vi "Dashboard Main.vi"() -> ()   [LabVIEW 2016]
uses:
  <vilib>/Rock Robotics/WPI/Camera/WPI_CameraExposure Values.ctl
  <vilib>/Rock Robotics/WPI/Camera/WPI_CameraWhite Balance Values.ctl
  <vilib>/Utility/miscctls.llb/LVRowAndColumnTypeDef.ctl
  <vilib>/event_ctls.llb/eventvkey.ctl
  <vilib>/Rock Robotics/Network Tables/NT Read Numeric Array.vi
  <vilib>/Rock Robotics/WPI/Dashboard/WPI_DashboardLogging Global.vi
  <vilib>/vision/NI_Vision_Development_Module.lvlib
panel:
  in  "Camera Settings 2":T3={"Exposure"=enum."Custom", "Exposure (%)"=0.0, "Brightness"=0, "White Balance"=enum."Custom", "Color Temp (K)"=0.0}
  out "Particle Reports (Pixels)":T4(array[cluster]) {"Orientation" format="%.2f"; "Dimensions"."Height" format="%.2f"; "Dimensions"."Width" format="%.2f"; "Center of Mass"."Y" format="%.2f"; "Center of Mass"."X" format="%.2f"; "Bounding Rect"."Bottom" format="%.2f"; "Bounding Rect"."Right" format="%.2f"; "Bounding Rect"."Top" format="%.2f"; "Bounding Rect"."Left" format="%.2f"; "Number of Holes" format="%.2f"; "Area" format="%.2f"}
  out "Detected and good":bool
  in  "Camera Settings Right":T5={"Frame Rate"=30, "Compression"=30, "Size"=1, "DB Camera Config"=FALSE} {"Frame Rate" scale=1.0..30.0; "Compression" scale=100.0..-1.0; "Size" items=["640x480", "320x240", "160x120"]}
  in  "Camera Name Right":string(combo)="No Camera Selection"
  out "Camera Info":cluster{"Mbps LED":bool, "Mbps":dbl, "fps":dbl} {"fps" format="%#.1g"; "Mbps" format="%#.1g"}
  in  "Camera Settings":T5={"Frame Rate"=30, "Compression"=30, "Size"=1, "DB Camera Config"=FALSE} {"Frame Rate" scale=1.0..30.0; "Compression" scale=100.0..-1.0; "Size" items=["640x480", "320x240", "160x120"]}
  in  "TCP":refnum<k5>
  in  "Rec Mode":enum32{"Stop", "Record", "Playback"}(radio)
  out "Robot IP":string
  out "Image Message":string="Timeout in Camera Communications"
  in  "Dashboard Tab":T6(tab)
  in  "Select Auto":string(combo)="Select Autonomous ..."
  out "NT Connection":bool
  out "MotorChart R":cluster{"Numeric":dbl, "Numeric":dbl}(graph)
  out "MotorChart L":cluster{"Numeric":dbl, "Numeric":dbl}(graph)
  out "MotorSliders R":cluster{"MotorSlide1":dbl, "MotorSlide2":dbl} {"MotorSlide2" scale=-1.0..1.0 scale format="%#_2e"; "MotorSlide1" scale=-1.0..1.0 scale format="%#_2e"}
  out "MotorSliders L":cluster{"MotorSlide1":dbl, "MotorSlide2":dbl} {"MotorSlide2" scale=-1.0..1.0 scale format="%#_2e"; "MotorSlide1" scale=-1.0..1.0 scale format="%#_2e"}
  out "Gyro":dbl(knob) scale=0.0..360.0
  out "JS1 Z":dbl(slide) scale=-1.0..1.0 scale format="%#_2e"
  out "JS1 Graph":cluster{"X":dbl, "Y":dbl}[](graph)
  out "JS1 Buttons":T7
  out "JS2 Z":dbl(slide) scale=-1.0..1.0 scale format="%#_2e"
  out "JS2 Graph":cluster{"X":dbl, "Y":dbl}[](graph)
  out "JS2 Buttons":T7
  out "Mode":T8(ring)=enum."Auto Disabled"
  in  "Observer Gain":dbl=0.5
  out "Detected":bool
  out "Camera Image Right":T9(plugin-control)
  in  "DB/String 9":string
  in  "DB/String 8":string
  in  "DB/String 7":string
  in  "DB/String 6":string
  in  "DB/String 5":string
  in  "DB/String 4":string
  in  "DB/String 3":string
  in  "DB/String 2":string
  in  "DB/String 1":string
  in  "DB/String 0":string
  in  "DB/Slider 0":dbl(slide) scale=0.0..5.0
  in  "DB/Slider 1":dbl(slide) scale=0.0..5.0
  in  "DB/Slider 2":dbl(slide) scale=0.0..5.0
  in  "DB/Slider 3":dbl(slide) scale=0.0..5.0
  out "DB/LED 3":bool
  out "DB/LED 2":bool
  out "DB/LED 1":bool
  out "DB/LED 0":bool
  in  "DB/Button 3":bool
  in  "DB/Button 2":bool
  in  "DB/Button 1":bool
  in  "DB/Button 0":bool caption="New Name"
  in  "Test Slider":dbl(slide) scale=0.0..100.0 scale format="%#_3g"
  in  "On/Off":bool caption="Solenoid"
  in  "Test Name":u16(ring) items=["Select the test to run..."]
  in  "Test Tree":string(tree)
  in  "Motor":cluster{"Value":dbl, "Enable":bool} {"Value" scale=-1.0..1.0 scale format="%#_3g"}
  out "Progress":T10 {"Test Progress" scale=0.0..100.0}
  in  "Rev/Fwd":cluster{"Forward":bool, "Reverse":bool}
  in  "Test Ring":u16(ring) items=["Monochrome", "Color"]
  out "Cmd Status":string
  in  "Execute Command":bool
  in  "Command Params":string[][](table)
  in  "Command Selection":i32(listbox)
  in  "CheckList":i32(listbox)
  out "Tree":string(tree)
  out "Camera Image":T9(plugin-control)
  out "Background":bool
  in  "Camera Name":string(combo)="Camera"
  # "HW"
  # "HW"
  # "Joysticks"
  # "Drive Motors"
  # "Front"
  # "Right"
  # "Left"
  # "Back"
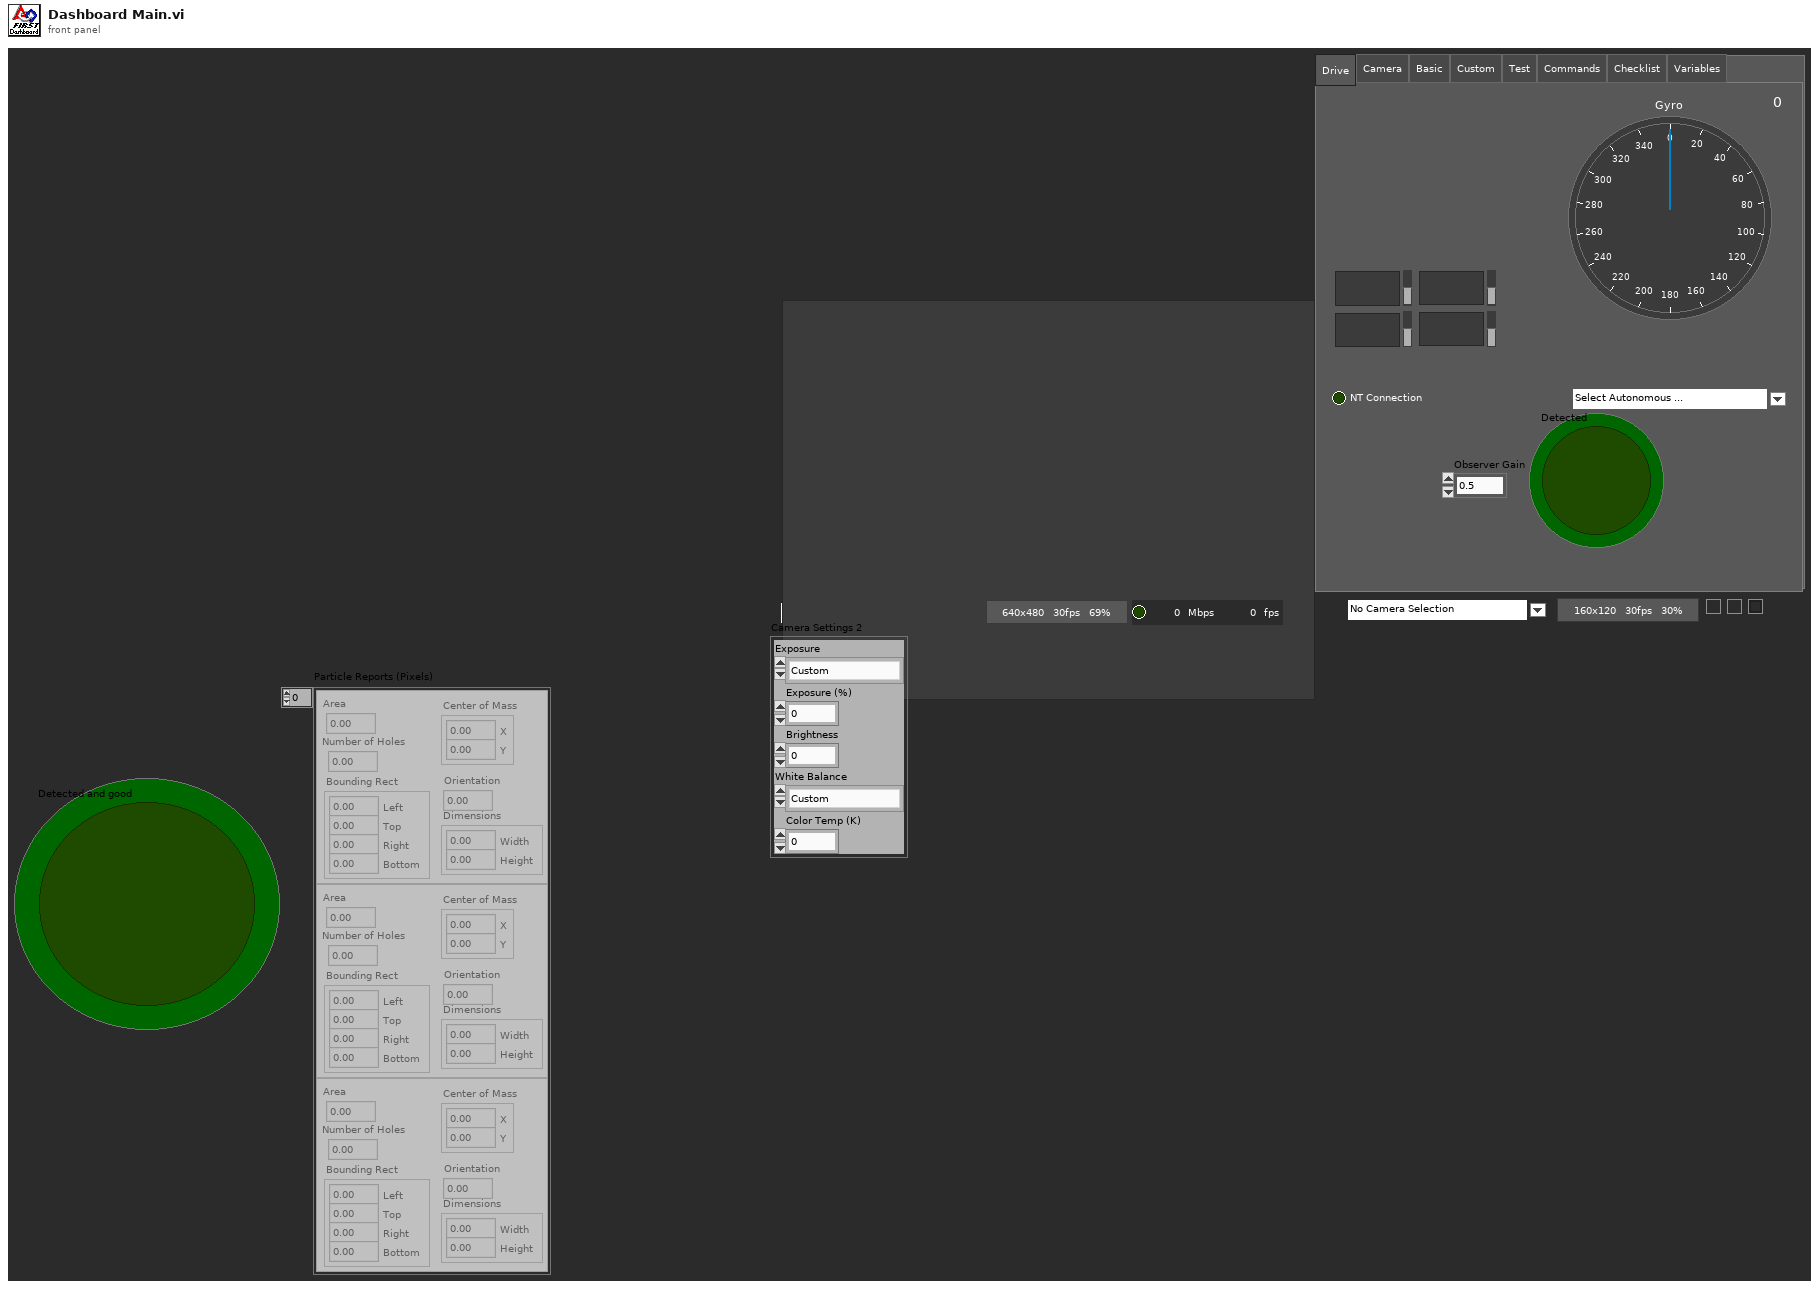
[diagram p1: front panel]
types:
  T1 = typedef "WPI_CameraExposure Values.ctl" = enum16{"Auto", "Flicker-free 50 Hz", "Flicker-free 60 Hz", "Hold current", "Custom"}
  T2 = typedef "WPI_CameraWhite Balance Values.ctl" = enum16{"Auto", "Fixed indoor", "Fixed outdoor 1", "Fixed outdoor 2", "Fixed fluorescent 1", "Fixed fluorescent 2", "Hold current", "Custom"}
  T3 = cluster{"Exposure":T1, "Exposure (%)":dbl, "Brightness":i32, "White Balance":T2, "Color Temp (K)":dbl}
  T4 = cluster{"Area":dbl, "Number of Holes":dbl, "Bounding Rect":cluster{"Left":dbl, "Top":dbl, "Right":dbl, "Bottom":dbl}, "Center of Mass":cluster{"X":dbl, "Y":dbl}, "Orientation":dbl, "Dimensions":cluster{"Width":dbl, "Height":dbl}}[]
  T5 = cluster{"Frame Rate":i32, "Compression":i32, "Size":u16, "DB Camera Config":bool}
  T6 = enum32{"Drive", "Camera", "Basic", "Custom", "Test", "Commands", "Checklist", "Variables"}
  T7 = cluster{bool, bool, bool, bool, bool, bool, bool, bool, bool, bool, bool, bool}
  T8 = enum8{"Tele-Op Disabled", "Tele-Op Enabled", "Auto Disabled", "Auto Enabled", "Test Disabled", "Test Enabled", "Disconnected", "No Code", "E-Stop"}
  T9 = typedef "IMAQ Image.ctl" = refnum<image>
  T10 = cluster{"Test Progress":u8, "Test Progress Text":string}
  T11 = typedef "Image Type" = u32
  T12 = cluster{"IDs":cluster{"RPC field ID":u16, "Unique ID":u16}, "String":string}
  T13 = enum32{"Drive", "Basic", "Custom", "Test", "Checklist", "Variables"}
  T14 = cluster{"Camera Image":refnum<vi>, "Dashboard Tab":refnum<vi>, "Background":refnum<vi>, "Rec Mode":refnum<vi>, "Test Slider":refnum<vi>, "On/Off ":refnum<vi>, "Test Ring":refnum<vi>, "Rev/Fwd":refnum<vi>, "Test Name":refnum<vi>, "Motor":refnum<vi>, "Progress":refnum<vi>, "CheckList":refnum<vi>, "Tree":refnum<vi>, "Test Tree":refnum<vi>, "Command Params":refnum<vi>, "Command Selection":refnum<vi>, "Execute Command":refnum<vi>, "Cmd Status":refnum<vi>, "Camera Settings":refnum<vi>, "Camera Name":refnum<vi>, "Camera Info":refnum<vi>, "Camera Settings Right":refnum<vi>, "Camera Name Right":refnum<vi>, "Camera Image Right":refnum<vi>}
  T15 = cluster{"Error Strings":string, "Disable Counts":cluster{u16, u16}, "Rail Faults":cluster{u16, u16, u16}, "Robot IP":string, "DB Mode":u8, "Event Info":cluster{"Name":string, "Type":u8, "Number":u16, "Replay":u8}}
  T16 = cluster{"Storage":cluster{"Disk Free":u64, "RAM Block":u32, "RAM free":u32}, "CPU Utilization":cluster{"CPU % ISR":sgl, "CPU % Time Crit":sgl, "CPU % Timed Str":sgl, "CPU % High":sgl, "CPU % Above":sgl, "CPU % Normal":sgl, "CPU % Low":sgl}, "CAN":cluster{"% Bus Utilization":sgl, "Bus Off Cnt":u32, "TX_FIFO Full Cnt":u32, "Receive Error Cnt":u8, "Transmit Error Cnt":u8}, "HID":cluster{"HID Outputs":u32, "Rumble Low":u16, "Rumble High":u16}[]}
  T17 = cluster{"Status bits":cluster{"Test Mode":bool, "Autonomous":bool, "Enabled":bool, "Code Start":bool, "Brownout":bool, "Reserved 2":bool, "Reserved 3":bool, "E-Stop":bool}, "Code Trace":cluster{"Disabled":bool, "TeleOp":bool, "Auto":bool, "Test":bool}, "Controller Type":enum16{"unknown", "cRIO", "roboRio"}, "Code?":enum16{"unknown", "noCode", "code"}, "Battery V":dbl}
  T18 = cluster{"Control Bits":cluster{"TestMode":bool, "Autonomous":bool, "Enabled":bool, "FMS Present":bool, bool, bool, bool, "E-Stop":bool}, "Team Station ":u8, "Countdown":sgl, "Joystick Values":cluster{"Axes":dbl[], "Buttons":bool[], "POVs":i16[]}[]}
  T19 = cluster{"Axes":dbl[], "Buttons":bool[], "POVs":i16[]}[]
  T20 = cluster{"Axes":dbl[], "Buttons":bool[], "POVs":i16[]}
  T21 = cluster{"Buttons[0]":bool, "Buttons[1]":bool, "Buttons[2]":bool, "Buttons[3]":bool, "Buttons[4]":bool, "Buttons[5]":bool, "Buttons[6]":bool, "Buttons[7]":bool, "Buttons[8]":bool, "Buttons[9]":bool, "Buttons[10]":bool, "Buttons[11]":bool}
  T22 = cluster{"Operation":enum16{"Update", "Clear"}, "Color Box":u32}[]
  T23 = typedef "eventvkey.ctl" = enum16{"ASCII", "Enter", "Return", "Shift", "Ctrl", "Alt", "Cmd", "Opt", "Caps", "NumLock", "Clear", "Break", "Up", "Down", "Left", "Right", "Insert", "Delete", "Home", "End", "PageUp", "PageDown", "Escape", "Help", "Pause", "ScrollLock", "F1", "F2", "F3", "F4", "F5", "F6", "F7", "F8", "F9", "F10", "F11", "F12", "F13", "F14", "F15", "F16", "F17", "F18", "F19", "F20", "F21", "F22", "F23", "F24", "Play", "VolumeUp", "VolumeDown", "Mute", "Two Byte Char"}
  T24 = cluster{"Image Size":bool, "Image Type":bool, "Pixel Value":bool, "ROI Information":bool, "Zoom Factor":bool}
  T25 = cluster{"Operation":enum16{"Update", "Clear"}, "Color Box":u32}
  T26 = typedef "LVRowAndColumnTypeDef.ctl" = cluster{"Row":i32, "Column":i32}
  T27 = cluster{"Shift":bool, "Ctrl":bool, "Alt":bool, "Cmd":bool, "Opt":bool}
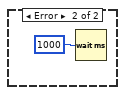
[diagram p3: hidden frame]
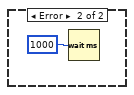
[diagram p4: hidden frame]
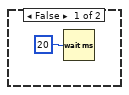
[diagram p5: hidden frame]
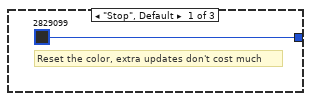
[diagram p6: hidden frame]
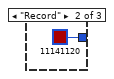
[diagram p7: hidden frame]
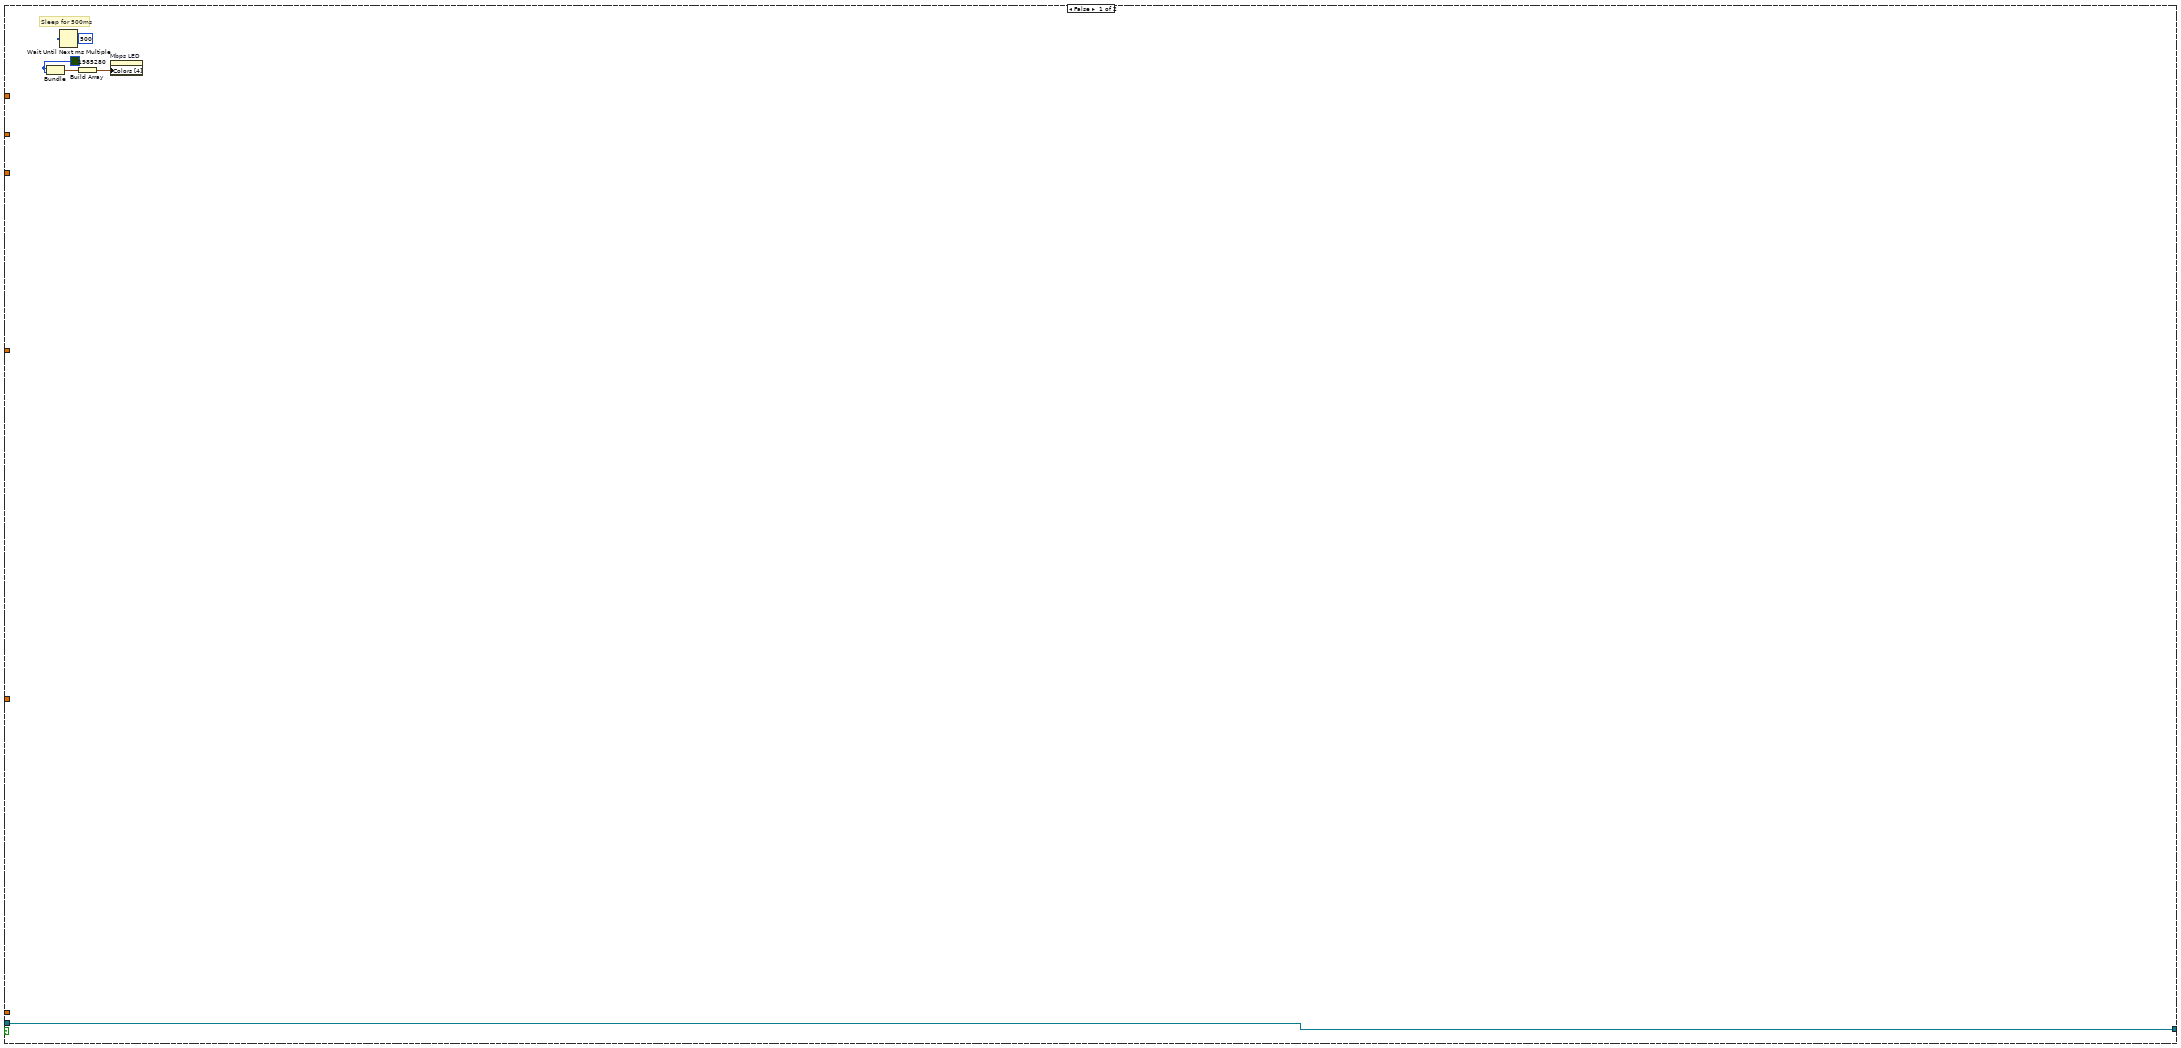
[diagram p9: hidden frame]
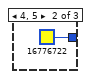
[diagram p11: hidden frame]
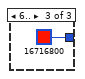
[diagram p12: hidden frame]
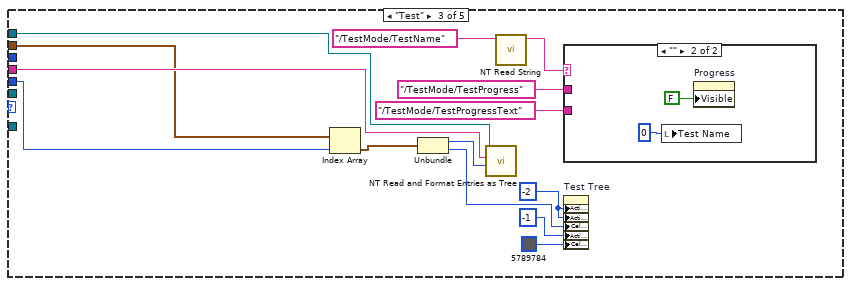
[diagram p14: hidden frame]
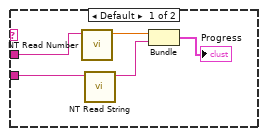
[diagram p15: hidden frame]
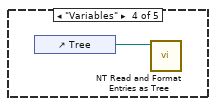
[diagram p16: hidden frame]
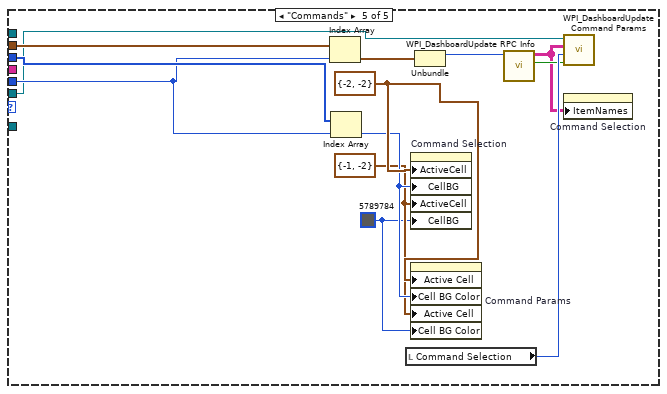
[diagram p17: hidden frame]
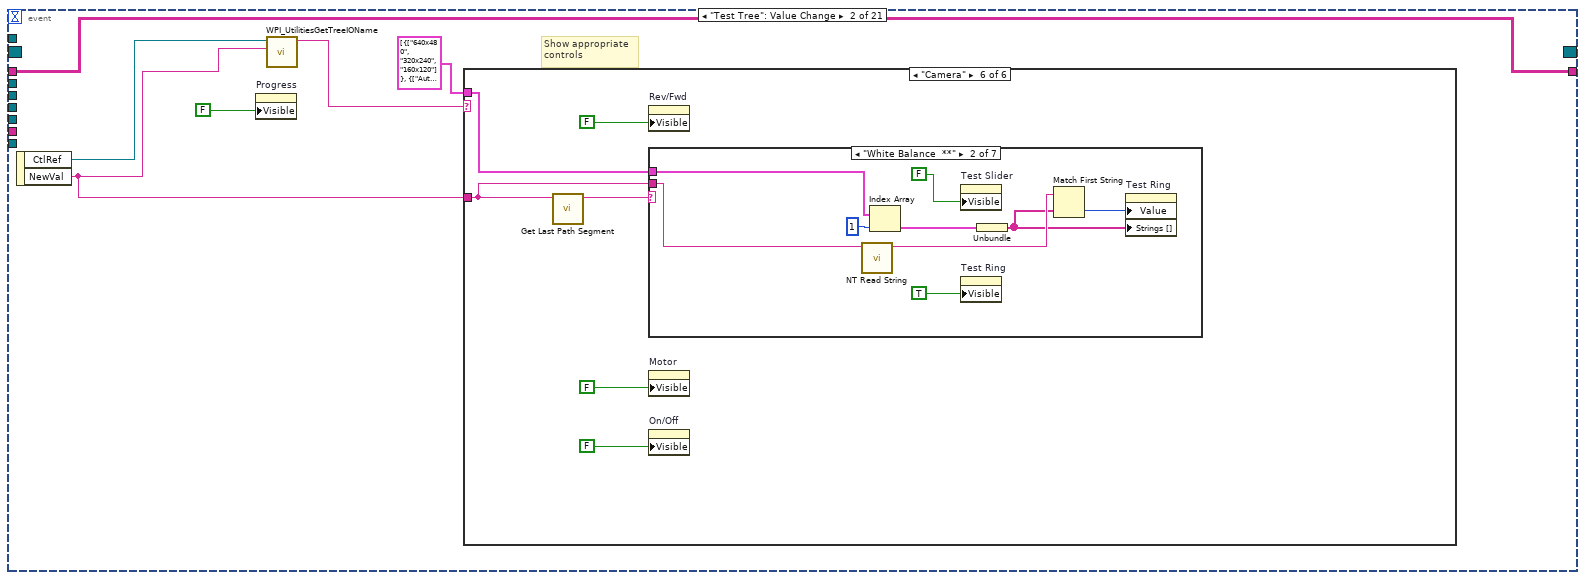
[diagram p18: hidden frame]
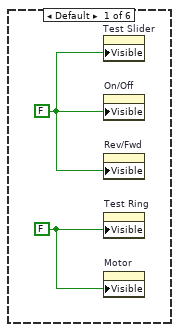
[diagram p19: hidden frame]
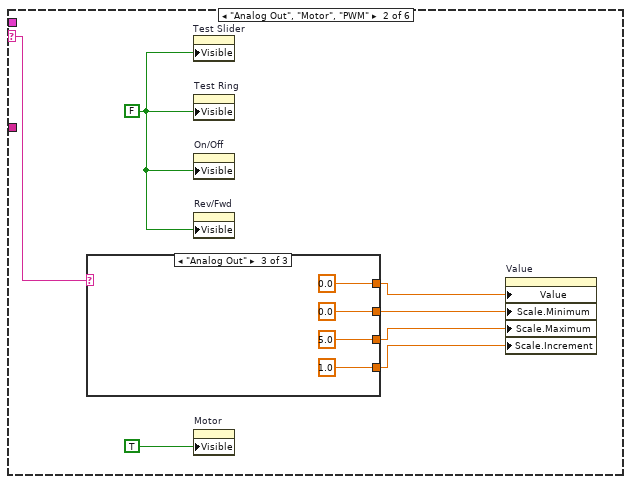
[diagram p20: hidden frame]
diagram:
  w10 = T11 4 items=["Grayscale (U8)", "Grayscale (I16)", "Grayscale (SGL)", "Complex (CSG)", "RGB (U32)", "HSL (U32)", "RGB (U64)"] ("Image Type")
  w26 = T12 {"IDs"={"RPC field ID"=0, "Unique ID"=0}, "String"=""}  # RPC Response
  w51 = 491  # min tab size
  w50 = 1.333  # min tab size
  w58 = enum32{"Stop", "Record", "Playback"}."Stop" ("Rec Mode")
  w33 = FALSE ("Visible")
  (unwired) "This VI has seven parallel loops for different tasks and a bit of initialization code that runs just once.\n\nTypical dashboard extensions only need to edit the panel. Adding new indicators or controls simply involves placing them on the panel in the Operations tab and naming them the same as the SmartDashboard variable on the robot\n\nIf the display needs to process the data before display, loop one is an example of doing that for the joysticks and motors.\n\nIf you want customize the video display or perform processing on it, loop two is where that takes place.\n\nOther loops should not need to be modified. They are pretty standard, and document the task they perform."  # Documentation
  w75 = T11 4 items=["Grayscale (U8)", "Grayscale (I16)", "Grayscale (SGL)", "Complex (CSG)", "RGB (U32)", "HSL (U32)", "RGB (U64)"] ("Image Type")
  # "Loop 2.5 Receive additional camera images from robot and display"
  # "Command Param Info"
  # "Started one, Unique ID holds\nresponse"
  # "Loop 7. Wait for DS connections"
  # "Basic debug and auto controls: Their data names are fixed, but\nthe displayed name, called a caption, can be changed directly or in\nrobot code such as shown in Begin."
  # "Controls for Test Mode, Camera Settings, etc."
  # "Additional UI Initialization"
  # "Loop 6. Animation for background of window during playback and record"
  # "Fires each time robot IP\nchanges, simulator does this"
  # "Fires each time window\ndocking changes."
  # "Collects all controls and indicators\nin the Basic and Custom tab.\nIf you need to bind additional controls,\nadd their references. You can extend the\nenum constant or use an integer."
  # "The remaining code below this line typically doesn't need to be modified."
  # "Loop 4. Process UI events related to test mode, checklist, and camera settings"
  # "Terminals of controls and indicators that are bound to the smart dashboard by name.\nYou can place the terminals anywhere you like and even read data from them.\nYou bind controls by adding the control reference to the array on the left. The subVI will\ndo this for the contents of a tab, and you can do it for individual items too, as shown with\nthe LED. To create get the reference, right-click and Create>>Reference."
  # "Loop 3. Wait until the robot response provides\n the Robot IP address.\nOnce known, bind controls and\nvariables with the same names."
  # "Loop 5. Adjusts placement onscreen, hides the titlebar, etc."
  # "Loop 1. Receive various data streams from Driver Station, update joystick, motors, and more complex displays that don't easily bind to variables."
  # "Loop 2. Receive camera images from robot, update Mbps, fps, and do any processing or display"
  n1 = control-ref of="Camera Settings"() -> (w19:refnum<vi>)
  n2 = control-ref of="Camera Name Right"() -> (w6:refnum<vi>)
  n3 = property class="VI"() -> ("Panel"=w65:refnum<vi>)  [unwired: 2 in, 2 out]
  n4 = control-ref of="Camera Name"() -> (w18:refnum<vi>)
  n5 = local write "Command Selection"(u16 0 ("milliseconds to wait")) -> ()
  n6 = property on="On/Off" class="Bool (strict)"("Visible"=w33) -> ()  [unwired: 2 in, 2 out]
  n7 = property on="Rev/Fwd" class="Clust (strict)"("Visible"=w33) -> ()  [unwired: 2 in, 2 out]
  n8 = property on="Motor" class="Clust (strict)"("Visible"=w33) -> ()  [unwired: 2 in, 2 out]
  n9 = property on="Progress" class="Clust (strict)"("Visible"=w33) -> ()  [unwired: 2 in, 2 out]
  n10 = property on="Test Ring" class="Ring (strict)"("Visible"=w33) -> ()  [unwired: 2 in, 2 out]
  n11 = while {
    tunnel: u16 1741 ("timeout ms (25000)") -> [w77]
    stop <- FALSE stop-if-true
    n12 = TCP Create Listener(10:w77) -> (0:w76:errorcluster, 3:w78:refnum<k5>)  [unwired: 4 in, 1 out]
    n13 = case shown="No Error" w76 {
      selector: w76 -> [w80 _]
      tunnel: w78 -> [w81 _]
      frame No Error {
        n14 = while {
          tunnel: w81 -> [w84]
          tunnel: w80 -> [w83]
          stop <- FALSE stop-if-true
          n15 = TCP Wait On Listener(8:w83, 11:w84) -> (0:w85:errorcluster, 4:w86:refnum<k5>)  [unwired: 2 in, 3 out]
          n16 = case shown="No Error" w85 {
            frame No Error {
            }
            frame Error {
              n17 = Wait (ms)(milliseconds to wait=u32 1000) -> ()  [unwired: 1 out]
            }
          }
          n18 = local write "TCP"(w86) -> ()
        }
      }
      frame Error {
        n19 = Wait (ms)(milliseconds to wait=u32 1000) -> ()  [unwired: 1 out]
      }
    }
  }
  n20 = local write "Rec Mode"(w58) -> ()
  n21 = global write "WPI_DashboardLogging Global.vi" "Recording"(w58) -> ()
  n22 = property class="Pnl"(reference=w65) -> ("Panes[]"=w66:refnum<vi>[])  [unwired: 1 in, 2 out]
  n23 = local write "Command Params"(string[][] [] ("Command Params")) -> ()
  n24 = local write "Dashboard Tab"(T6."Drive" ("Dashboard Tab")) -> ()
  n25 = call "Handle Camera Configuration.vi"("CameraNameRef"=w18, "Camera File Name"="Left", "ClusterRef"=w19) -> ()  [unwired: 9 in]
  n26 = call "IMAQ Create"("Image Name"="Dashboard Image", "Image Type"=w75) -> ("New Image"=w73:T9, "error out"=w72:errorcluster)  [unwired: 2 in, 1 out]
  n27 = Index Array(array=w66) -> (element=w64:refnum<vi>)  [unwired: 1 in]
  n28 = call "IMAQ Create"("Image Name"="Dashboard ImageRight", "Image Type"=w10) -> ("New Image"=w9:T9, "error out"=w8:errorcluster)  [unwired: 2 in, 1 out]
  n29 = while {
    tunnel: w73 -> [w95]
    tunnel: w72 -> [_]
    tunnel: [w96] -> _
    i -> [w96]
    stop <- FALSE stop-if-true
    n30 = flat-sequence {
      tunnel: w95 -> [w104]
      tunnel: [w104] -> w94
      tunnel: [w102] -> w93
      tunnel: [w98] -> w92
      tunnel: [w99] -> w91
      tunnel: [w99] -> w90
      tunnel: [w98] -> w89
      tunnel: w94 -> [w120]
      tunnel: w93 -> [w111]
      tunnel: w92 -> [w110]
      tunnel: w91 -> [w109]
      tunnel: w90 -> [w108]
      tunnel: w89 -> [w107]
      frame #0 {
        n31 = call-poly <vilib>:"NT Read Value.vi"("Name"="Y Latency") -> ("Numeric"=w99:dbl)  [unwired: 9 in, 1 out]
        n32 = call-poly <vilib>:"NT Read Value.vi"("Name"="X Latency") -> ("Numeric"=w98:dbl)  [unwired: 9 in, 1 out]
        n33 = call-poly <vilib>:"NT Read Value.vi"("Name"="Navx Yaw Latency") -> ("Numeric"=w102:dbl)  [unwired: 9 in, 1 out]
      }
      frame #1 {
        # "Optionally read the DB image,\nlog, or retrieve images from a\nlogged match"
        n34 = local read "Rec Mode"() -> (w116:enum32{"Stop", "Record", "Playback"})
        n35 = local read "Robot IP"() -> (w115:string)
        n36 = call <vilib>:"WPI_CameraRead MJPG for Dashboard.vi"("Camera Settings"="Camera Settings", "Camera Settings 2"="Camera Settings 2", "Rec Mode"=w116, "Robot IP"=w115, "Camera Name"="Camera Name", "Refnum in"=w120) -> ("Active"=w118:bool, "Refnum out"=w119:T9, "FPS"=w117:dbl, "Bandwidth (Mbps)"=w114:dbl)  [unwired: 2 in]
        n37 = case shown="True" w118 {
          tunnel: w119 -> [w121 w144]
          tunnel: w114 -> [_ w141]
          tunnel: w117 -> [_ w142]
          tunnel: [w121 w135] -> w112
          tunnel: w111 -> [_ w129]
          tunnel: w110 -> [_ w131]
          tunnel: w109 -> [_ w130]
          tunnel: w108 -> [_ w133]
          tunnel: w107 -> [_ w132]
          frame False {
            w123 = u32 1985280 ("Color Box")
            # "Sleep for 500ms"
            n38 = Bundle("Color Box"=w123, "Color Box"=w123) -> (w124:cluster{"Color Box":u32, "Color Box":u32})  [unwired: 1 out]
            n39 = Wait Until Next ms Multiple(millisecond multiple=u32 500) -> ()  [unwired: 1 out]
            n40 = Build Array(w124) -> (w122:cluster{"Color Box":u32, "Color Box":u32}[])
            n41 = property on="Mbps LED" class="Bool (strict)"("Colors [4]"=w122) -> ()  [unwired: 2 in, 2 out]
          }
          frame True {
            # "im sorry"
            # "update motors & other I/O or global variables"
            # "Reconfigure camera image size and any\nother settings that need to change during\nthe match?"
            # "Here is where you would annotate,\npossibly process, and display the image"
            # "Update Mbps LED"
            n42 = case shown="Default" w141 {
              tunnel: [u32 6618880 ("Color Box") u32 16776722 ("Color Box") u32 16716800 ("Color Box")] -> w145
              frame Default {
              }
              frame 4, 5 {
              }
              frame 6.. {
              }
            }
            n43 = call "IMAQ Clear Overlay"("Image"=w144) -> ("error out"=w147:errorcluster, "Image Out"=w135:T9)  [unwired: 2 in, 7 out]
            n44 = Bundle(FALSE, "Bandwidth (Mbps)"=w141, "FPS"=w142) -> (→"Camera Info":cluster{bool, "Bandwidth (Mbps)":dbl, "FPS":dbl})  [unwired: 1 in]
            n45 = Unbundle By Name(w147) -> ("status"=w148:bool)
            n46 = call "vision v4.vi"("Image In"=w135) -> ("Image Out"=w134:T9)  [unwired: 25 in, 1 out]
            n47 = call "IMAQ Particle Analysis Report"("Connectivity 4/8 (8)"=TRUE, "Image"=w134) -> ("Particle Reports (Pixels)"=w128:T4)  [unwired: 4 in, 5 out]
            n48 = property on="Image Message" class="Str"("Visible"=w148) -> ()  [unwired: 2 in, 2 out]
            n49 = call "Eliminate Wrong Target.vi"("Particle Reports (Pixels)"=w128) -> ("Target Particle Reports (Pixels)"=w127:T4)
            "Particle Reports (Pixels)" <- w127
            n50 = Array Size(array=w127) -> (size(s)=w126:i32)
            n51 = Bundle("Color Box"=w145, "Color Box"=w145) -> (w146:cluster{"Color Box":u32, "Color Box":u32})  [unwired: 1 out]
            n52 = Equal?(x=w126, y=2) -> (x = y?=w136:bool)
            "Detected and good" <- w136
            "Detected" <- w136
            n53 = case shown="True" w136 {
              tunnel: w127 -> [_ w156]
              tunnel: w129 -> [_ _]
              tunnel: w133 -> [_ _]
              tunnel: w132 -> [_ _]
              tunnel: w131 -> [_ w154]
              tunnel: w130 -> [_ w153]
              tunnel: w129 -> [_ w152]
              frame False {
              }
              frame True {
                # "Estimate Y"
                # "Estimate X"
                n54 = call "Goal Position From Robot and Camera.vi"("Navx Yaw"=w152, "Pose Y"=w153, "Pose X"=w154, "Targets"=w156) -> ("Goal Y"=w150:dbl, "Goal X"=w151:dbl)
                n55 = feedback #1(w151) -> (w155:dbl)
                n56 = Subtract(x=w151, y=w155) -> (x-y=w158:dbl)
                n57 = Multiply(x=w158, y="Observer Gain") -> (x*y=w163:dbl)
                n58 = feedback #2(w150) -> (w157:dbl)
                n59 = Subtract(x=w150, y=w157) -> (x-y=w159:dbl)
                n60 = Multiply(x="Observer Gain", y=w159) -> (x*y=w162:dbl)
                n61 = Add(x=w163, y=w155) -> (x+y=w161:dbl)
                n62 = feedback-in #1(w161) -> ()
                n63 = Add(x=w162, y=w157) -> (x+y=w160:dbl)
                n64 = feedback-in #2(w160) -> ()
                n65 = call-poly <vilib>:"NT Write Value.vi"("Numeric"=w161, "Name"="Goal X") -> ()  [unwired: 9 in, 1 out]
                n66 = call-poly <vilib>:"NT Write Value.vi"("Numeric"=w160, "Name"="Goal Y") -> ()  [unwired: 9 in, 1 out]
              }
            }
            n67 = Build Array(w146) -> (w143:cluster{"Color Box":u32, "Color Box":u32}[])
            n68 = property on="Mbps LED" class="Bool (strict)"("Colors [4]"=w143) -> ()  [unwired: 2 in, 2 out]
          }
        }
        "Camera Image" <- w112
      }
    }
  }
  n69 = control-ref of="Dashboard Tab"() -> (w56:refnum<vi>)
  n70 = control-ref of="Camera Settings Right"() -> (w7:refnum<vi>)
  n71 = while {
    tunnel: w64 -> [w170]
    i -> [w173]
    stop <- FALSE stop-if-true
    n72 = Wait (ms)(milliseconds to wait=u32 100) -> ()  [unwired: 1 out]
    n73 = case shown="\"Playback\"" "Rec Mode" {
      tunnel: w173 -> [_ _ w188]
      tunnel: [u32 2829099 ("Base Color") u32 11141120 ("Target Color") w177] -> w169
      frame "Stop", Default {
        # "Reset the color, extra updates don't cost much"
      }
      frame "Record" {
      }
      frame "Playback" {
        # "Playback"
        n74 = Quotient & Remainder(x=w188, y=u32 50 ("milliseconds to wait")) -> (x-y*floor(x/y)=w184:u32)  [unwired: 1 out]
        n75 = Divide(x=w184, y=u32 50 ("milliseconds to wait")) -> (x/y=w181:dbl)
        n76 = Multiply(x=6.283185307179586, y=w181) -> (x*y=w186:dbl)
        n77 = Sine(x=w186) -> (sin(x)=w185:dbl)
        n78 = Absolute Value(x=w185) -> (abs(x)=w178:dbl)
        n79 = call "Interpolate RGB Color.vi"("Proportion"=w178, "Target Color"=u32 30976, "Base Color"=u32 2829099) -> ("Result Color"=w177:u32)  [unwired: 8 in]
      }
    }
    n80 = property class="Pane"(reference=w170, "PaneColor"=w169) -> ()  [unwired: 1 in, 2 out]
  }
  n81 = while {
    tunnel: w9 -> [w199]
    tunnel: w8 -> [_]
    tunnel: [w193] -> _
    i -> [w193]
    stop <- FALSE stop-if-true
    n82 = local read "Rec Mode"() -> (w197:enum32{"Stop", "Record", "Playback"})
    n83 = local read "Robot IP"() -> (w198:string)
    n84 = call <vilib>:"WPI_CameraRead MJPG for Dashboard.vi"("Camera Settings"="Camera Settings Right", "Rec Mode"=w197, "Robot IP"=w198, "Camera Name"="Camera Name Right", "Refnum in"=w199) -> ("Active"=w192:bool, "Refnum out"=w195:T9, "FPS"=w190:dbl, "Bandwidth (Mbps)"=w191:dbl)  [unwired: 3 in]
    n85 = case shown="False" w192 {
      tunnel: w195 -> [w201 w203]
      tunnel: w191 -> [_ _]
      tunnel: w190 -> [_ _]
      tunnel: [w201 w203] -> w189
      frame False {
        n86 = Wait Until Next ms Multiple(millisecond multiple=u32 500) -> ()  [unwired: 1 out]
      }
      frame True {
      }
    }
    "Camera Image Right" <- w189
  }
  n87 = call <vilib>:"Get Tab Control Refs.vi"("Page Index"=T13."Custom" ("Dashboard Tab"), "TabControl in"=w56) -> ("ControlsOnPage"=w55:refnum<vi>[])  [unwired: 9 in]
  n88 = call <vilib>:"Get Tab Control Refs.vi"("Page Index"=T13."Basic" ("Dashboard Tab"), "TabControl in"=w56) -> ("ControlsOnPage"=w14:refnum<vi>[])  [unwired: 9 in]
  n89 = Create User Event(user event datatype=w26) -> (user event=w22:refnum<user-event>)  [unwired: 1 in, 1 out]
  n90 = call "Handle Camera Configuration.vi"("CameraNameRef"=w6, "Camera File Name"="Right", "ClusterRef"=w7) -> ()  [unwired: 9 in]
  n91 = call <vilib>:"NT Write String.vi"("String"="Select Auto", "Name"="Auto Selector") -> ()  [unwired: 9 in, 1 out]
  n92 = Build Array (concatenate)(w14, w55) -> (w54:refnum<vi>[])
  n93 = Obtain Notifier(name (unnamed)="Robot IP Update", notification data type="IP Addr" ("name (unnamed)")) -> (notifier out=w32:refnum<notifier>)  [unwired: 2 in, 2 out]
  n94 = control-ref of="CheckList"() -> (w44:refnum<vi>)
  n95 = call "Initialize Camera and CheckList.vi"("ListBox in"=w44) -> ()  [unwired: 11 in]
  n96 = register-events(refnum<vi> refnum, w22) -> (reference out=w62:refnum<event-registration>, error out=w61:errorcluster)  [unwired: 2 in]
  n97 = control-ref of="Rec Mode"() -> (w39:refnum<vi>)
  n98 = control-ref of="Command Selection"() -> (w25:refnum<vi>)
  n99 = control-ref of="Camera Settings Right"() -> (w3:refnum<vi>)
  n100 = control-ref of="Camera Image Right"() -> (w1:refnum<vi>)
  n101 = control-ref of="Camera Name Right"() -> (w2:refnum<vi>)
  n102 = control-ref of="Execute Command"() -> (w27:refnum<vi>)
  n103 = control-ref of="Command Params"() -> (w28:refnum<vi>)
  n104 = control-ref of="Camera Image"() -> (w53:refnum<vi>)
  n105 = control-ref of="Camera Settings"() -> (w17:refnum<vi>)
  n106 = control-ref of="Dashboard Tab"() -> (w52:refnum<vi>)
  n107 = control-ref of="Tree"() -> (w43:refnum<vi>)
  n108 = control-ref of="Test Tree"() -> (w42:refnum<vi>)
  n109 = control-ref of="Camera Name"() -> (w16:refnum<vi>)
  n110 = control-ref of="Background"() -> (w48:refnum<vi>)
  n111 = control-ref of="Camera Info"() -> (w15:refnum<vi>)
  n112 = control-ref of="Cmd Status"() -> (w21:refnum<vi>)
  n113 = control-ref of="On/Off"() -> (w37:refnum<vi>)
  n114 = control-ref of="Test Name"() -> (w41:refnum<vi>)
  n115 = control-ref of="Test Slider"() -> (w38:refnum<vi>)
  n116 = control-ref of="Rev/Fwd"() -> (w35:refnum<vi>)
  n117 = control-ref of="Motor"() -> (w40:refnum<vi>)
  n118 = control-ref of="Progress"() -> (w34:refnum<vi>)
  n119 = control-ref of="Test Ring"() -> (w36:refnum<vi>)
  n120 = vi-ref "Playback Controls.vi"() -> (w63:refnum<vi>)
  n121 = control-ref of="Command Params"() -> (w20:refnum<vi>)
  n122 = Bundle("Camera Image"=w53, "Dashboard Tab"=w52, "Background"=w48, "Rec Mode"=w39, "Test Slider"=w38, "On/Off"=w37, "Test Ring"=w36, "Rev/Fwd"=w35, "Test Name"=w41, "Motor"=w40, "Progress"=w34, "CheckList"=w44, "Tree"=w43, "Test Tree"=w42, "Command Params"=w28, "Command Selection"=w25, "Execute Command"=w27, "Cmd Status"=w21, "Camera Settings"=w17, "Camera Name"=w16, "Camera Info"=w15, "Camera Settings Right"=w3, "Camera Name Right"=w2, "Camera Image Right"=w1) -> (w45:T14)  [unwired: 1 in]
  n123 = Bundle("min tab size"=w51, "min tab size"=w50) -> (w49:cluster{"min tab size":i32, "min tab size":dbl})  [unwired: 1 in]
  n124 = control-ref of="Test Tree"() -> (w67:refnum<vi>)
  n125 = property class="VI" props=["Front Panel.Closeable"]() -> (reference out=w57:refnum<vi>)  [unwired: 2 in, 2 out]
  n126 = Obtain Notifier(name (unnamed)="Window Mode", notification data type=TRUE) -> (notifier out=w31:refnum<notifier>)  [unwired: 2 in, 2 out]
  n127 = call "Adjust Dashboard Window.vi"("Sizing Refnums"=w45, "Size Constraints"=w49, "VI"=w57, "WIn Mode"=w31) -> ()  [unwired: 8 in]
  n128 = while {
    tunnel: w54 -> [w215]
    tunnel: w32 -> [w213]
    tunnel: [w211] -> _
    tunnel: u32 1000 ("milliseconds to wait") -> [w210]
    tunnel: w22 -> [w204]
    i -> [w211]
    stop <- FALSE stop-if-true
    n129 = Wait on Notification(notifier=w213, timeout in ms (-1)=w210) -> (notification=w212:string, timed out?=w208:bool)  [unwired: 2 in, 2 out]
    n130 = local read "Rec Mode"() -> (w206:enum32{"Stop", "Record", "Playback"})
    n131 = Equal?(x=w206, y=u16 2 ("Rec Mode")) -> (x = y?=w207:bool)
    n132 = Compound Arithmetic op=OR(invert w208, w207) -> (w209:bool)
    n133 = case shown="True" w209 {
      tunnel: w215 -> [_ w218]
      tunnel: w212 -> [_ w217]
      tunnel: w204 -> [_ w216]
      frame False {
      }
      frame True {
        n134 = call <vilib>:"Bind Controls to SmartDashboard.vi"("RPC ref"=w216, "Bound Control Refs"=w218, "Server IP Address"=w217) -> ()  [unwired: 9 in]
      }
    }
  }
  n135 = while {
    tunnel: [w228] -> _
    tunnel: w32 -> [w222]
    tunnel: w31 -> [w219]
    i -> [w228]
    stop <- FALSE stop-if-true
    n136 = call <vilib>:"WPI_DashboardRetrieveStatusInfo.vi"("Binding Refnum"=w222, "Window Mode Notifier"=w219, "TCP Cnx"="TCP") -> ("Power and Errors"=w223:T15, "Robot Metrics"=w226:T16, "Status Info"=w227:T17, "Control Info"=w224:T18, "Robot Mode"=w221:T8, "Process?"=w225:bool)  [unwired: 3 in]
    "Mode" <- w221
    n137 = case shown="True" w225 {
      tunnel: w227 -> [_ w254]
      tunnel: w226 -> [_ w253]
      tunnel: w224 -> [_ w252]
      tunnel: w223 -> [_ w251]
      tunnel: w221 -> [_ _]
      frame False {
        n138 = Wait (ms)(milliseconds to wait=u32 20) -> ()  [unwired: 1 out]
      }
      frame True {
        # "swap motors to match\ncharts and include battery"
        n139 = Unbundle By Name(w252) -> ("Joystick Values"=w242:T19)  [unwired: 1 out]
        n140 = Unbundle By Name(w254) -> ()  [unwired: 2 out]
        n141 = Unbundle By Name(w253) -> ()  [unwired: 1 out]
        n142 = Unbundle By Name(w251) -> ("Robot IP"=→"Robot IP":string)
        n143 = Index Array(array=w242) -> (element #1=w241:T20, element #2=w237:T20)  [unwired: 2 in]
        n144 = call "Prepare Joystick Data for Displays.vi"("Joystick Values"=w241) -> ("Buttons"=→"JS1 Buttons":T21, "Z Axis"=→"JS1 Z":dbl, "Cartesian Data"=→"JS1 Graph":cluster{"X axis":dbl, "X axis":dbl}[])  [unwired: 8 in]
        n145 = call "Prepare Joystick Data for Displays.vi"("Joystick Values"=w237) -> ("Buttons"=→"JS2 Buttons":T21, "Z Axis"=→"JS2 Z":dbl, "Cartesian Data"=→"JS2 Graph":cluster{"X axis":dbl, "X axis":dbl}[])  [unwired: 8 in]
        n146 = call-poly <vilib>:"NT Read Value.vi"("Name"="RobotDrive Motors") -> ("Numeric Array"=w232:dbl[])  [unwired: 9 in, 1 out]
        n147 = Index Array(array=w232, index #1=1, index #4=0) -> (element #1=w246:dbl, element #2=w247:dbl, element #3=w245:dbl, element #4=w250:dbl)  [unwired: 2 in]
        n148 = Bundle("Numeric"=w245, "Numeric"=w246) -> (→"MotorChart R" →"MotorSliders R":cluster{"Numeric":dbl, "Numeric":dbl})  [unwired: 1 in]
        n149 = Bundle("Numeric"=w247, "Numeric"=w250) -> (→"MotorChart L" →"MotorSliders L":cluster{"Numeric":dbl, "Numeric":dbl})  [unwired: 1 in]
      }
    }
  }
  n150 = while {
    tunnel: [w264] -> _
    tunnel: w67 -> [w263]
    tunnel: w63 -> [w262]
    tunnel: w62 -> [w261]
    tunnel: w61 -> [_]
    tunnel: w57 -> [w260]
    tunnel: w22 -> [w259]
    tunnel: w20 -> [w258]
    shift-right: [w257] -> _
    shift-left: _ -> [w256]
    tunnel: w14 -> [w255]
    i -> [w264]
    stop <- FALSE stop-if-true
    n151 = event shown="[0] Timeout" {
      selector: w261 -> [_ _ _ _ _ _ _ _ _ _ _ _ _ _ _ _ _ _ _ _ _]
      dyn-events: [_ _ _ _ _ _ _ _ _ _ _ _ _ _ _ _ w520 _ _ _ _] -> _
      timeout: u32 60 ("milliseconds to wait") -> [_ _ _ _ _ _ _ _ _ _ _ _ _ _ _ _ _ _ _ _ _]
      tunnel: w263 -> [w276 _ _ _ _ _ _ _ _ _ _ _ _ _ _ _ _ _ _ _ _]
      tunnel: "Test Tree" -> [_ _ _ _ _ _ _ _ _ _ _ w487 w495 w497 w501 w509 _ _ _ _ _]
      tunnel: w262 -> [_ _ _ _ _ _ _ _ _ _ _ _ _ _ _ _ w522 _ w540 _ _]
      tunnel: w260 -> [_ _ _ _ _ _ _ _ _ _ _ _ _ _ _ _ w518 _ _ _ _]
      tunnel: w259 -> [_ _ _ _ _ _ _ _ _ _ _ _ _ _ _ _ w514 _ _ _ _]
      tunnel: w258 -> [w271 _ _ _ _ _ w438 _ _ _ _ _ _ _ _ _ _ _ _ _ _]
      tunnel: [w270 w315 w417 w422 w431 w435 w436 w445 w455 w462 w474 w486 w493 w496 w500 w508 w513 w535 w537 w541 w552] -> w257
      tunnel: w256 -> [w270 w315 w417 w422 w431 w435 w436 _ _ w462 w474 w486 w493 w496 w500 w508 w513 w535 w537 w541 w552]
      tunnel: w255 -> [w268 _ _ _ _ _ _ _ _ _ _ _ _ _ _ _ _ _ _ _ _]
      event Timeout {
        n152 = event-data() -> ()  [unwired: 1 in, 1 out]
        n153 = call <vilib>:"Connextion Info.vi"() -> ("Connected"=→"NT Connection":bool)  [unwired: 10 in, 1 out]
        n154 = local read "Mode"() -> (w273:T8)
        n155 = case shown="\"Basic\"" "Dashboard Tab" {
          tunnel: w276 -> [_ _ w292 _ _]
          tunnel: "/TestMode/Automatic/" ("Name Pattern") -> [_ _ w291 _ _]
          tunnel: T22 [{"Operation"=enum."Clear", "Color Box"=14013909}, {"Operation"=enum."Clear", "Color Box"=14013909}, {"Operation"=enum."Clear", "Color Box"=14013909}, {"Operation"=enum."Clear", "Color Box"=14013909}, {"Operation"=enum."Update", "Color Box"=14013909}, {"Operation"=enum."Update", "Color Box"=16777215}, {"Operation"=enum."Clear", "Color Box"=14013909}, {"Operation"=enum."Clear", "Color Box"=14013909}, {"Operation"=enum."Clear", "Color Box"=14013909}] -> [_ _ w284 _ w308]
          tunnel: w273 -> [_ _ w283 _ w307]
          tunnel: u32[] [15790320, 15790320, 15790320, 15790320, 16777215, 16777215, 15790320, 15790320, 15790320] -> [_ _ _ _ w313]
          tunnel: w271 -> [_ _ _ _ w301]
          tunnel: w268 -> [_ w278 _ _ _]
          frame "Custom", Default {
          }
          frame "Basic" {
            n156 = call <vilib>:"WPI_DashboardUpdateNames.vi"("Controls on Tab"=w278) -> ()  [unwired: 11 in]
          }
          frame "Test" {
            w290 = -2 ("Active Item:Row Number")
            n157 = Index Array(array=w284, index=w283) -> (element=w285:T25)
            n158 = Unbundle(w285) -> ("Operation"=w286:enum16{"Update", "Clear"}, "Color Box"=w287:u32)
            n159 = call <vilib>:"NT Read and Format Entries as Tree.vi"("Operation"=w286, "Name Pattern"=w291, "Tree Refnum"=w292) -> ()  [unwired: 7 in, 2 out]
            n160 = call <vilib>:"NT Read String.vi"("Name"="/TestMode/TestName") -> ("String"=w281:string)  [unwired: 9 in, 1 out]
            n161 = case shown="\"\"" w281 {
              tunnel: "/TestMode/TestProgress" ("Name") -> [w294 _]
              tunnel: "/TestMode/TestProgressText" ("Name") -> [w293 _]
              frame Default {
                n162 = call <vilib>:"NT Read Number.vi"("Name"=w294) -> ("Numeric"=w295:dbl)  [unwired: 9 in, 1 out]
                n163 = call <vilib>:"NT Read String.vi"("Name"=w293) -> ("String"=w296:string)  [unwired: 9 in, 1 out]
                n164 = Bundle("Numeric"=w295, "String"=w296) -> (→"Progress":cluster{"Numeric":dbl, "String":string})  [unwired: 1 in]
              }
              frame "" {
                n165 = local write "Test Name"(u16 0) -> ()
                n166 = property on="Progress" class="Clust (strict)"("Visible"=FALSE) -> ()  [unwired: 2 in, 2 out]
              }
            }
            n167 = property on="Test Tree" class="Tree (strict)"("Active Item Row Number"=w290, "ActiveColNum"=w290, "CellBG"=w287, "Active Item Row Number"=-1 ("Active Item:Row Number"), "CellBG"=u32 5789784 ("Color Box")) -> ()  [unwired: 2 in, 2 out]
          }
          frame "Variables" {
            n168 = control-ref of="Tree"() -> (w300:refnum<vi>)
            n169 = call <vilib>:"NT Read and Format Entries as Tree.vi"("Tree Refnum"=w300) -> ()  [unwired: 9 in, 2 out]
          }
          frame "Commands" {
            w309 = u32 5789784 ("Color Box")
            w310 = T26 {"Row"=-1, "Column"=-2} ("Active Cell:Active Cell")
            w312 = T26 {"Row"=-2, "Column"=-2} ("Active Cell:Active Cell")
            n170 = Index Array(array=w308, index=w307) -> (element=w306:T25)
            n171 = Index Array(array=w313, index=w307) -> (element=w311:u32)
            n172 = local read "Command Selection"() -> (w304:i32)
            n173 = property on="Command Selection" class="MCListbox (strict)"("ActiveCell"=w312, "CellBG"=w311, "ActiveCell"=w310, "CellBG"=w309) -> ()  [unwired: 2 in, 2 out]
            n174 = property on="Command Params" class="Tbl (strict)"("Active Cell"=w312, "Cell BG Color"=w311, "Active Cell"=w310, "Cell BG Color"=w309) -> ()  [unwired: 2 in, 2 out]
            n175 = Unbundle(w306) -> ("Operation"=w305:enum16{"Update", "Clear"})  [unwired: 1 out]
            n176 = call <vilib>:"WPI_DashboardUpdate RPC Info.vi"("Operation"=w305) -> ("update"=w303:bool, "commands"=w302:string[][])  [unwired: 9 in]
            n177 = call <vilib>:"WPI_DashboardUpdate Command Params.vi"("Update"=w303, "NewVal"=w304, "Commands"=w302, "Param Tbl"=w301) -> ()  [unwired: 7 in, 1 out]
            n178 = property on="Command Selection" class="MCListbox (strict)"("ItemNames"=w302) -> ()  [unwired: 2 in, 2 out]
          }
        }
      }
      event "Test Tree": Value Change {
        # "Show appropriate\ncontrols"
        n179 = event-data() -> ("CtlRef"=w318:refnum<vi>, "NewVal"=w316:string)  [unwired: 1 in]
        n180 = property on="Progress" class="Clust (strict)"("Visible"=FALSE) -> ()  [unwired: 2 in, 2 out]
        n181 = call <vilib>:"WPI_UtilitiesGetTreeIOName.vi"("NewVal"=w316, "TreeControl in"=w318) -> ("I/O Name"=w319:string)  [unwired: 9 in]
        n182 = case shown="\"Camera\"" w319 {
          selector: w319 -> [_ w326 _ w348 w357 _]
          tunnel: w316 -> [_ _ w345 w347 _ w364]
          tunnel: cluster{string[]}[] [{["640x480", "320x240", "160x120"]}, {["Auto", "Fixed indoor", "Fixed outdoor 1", "Fixed outdoor 2", "Fixed fluorescent 1", "Fixed fluorescent 2", "Hold current"]}, {["Auto", "Flicker-free 50 Hz", "Flicker-free 60 Hz", "Hold current"]}, {["None", "Prioritize frame rate", "Prioritize image quality"]}, {["Monochrome", "Color"]}] -> [_ _ _ _ _ w363]
          frame Default {
            w321 = FALSE ("Visible")
            w320 = FALSE ("Visible")
            n183 = property on="Test Slider" class="Slide (strict)"("Visible"=w321) -> ()  [unwired: 2 in, 2 out]
            n184 = property on="On/Off" class="Bool (strict)"("Visible"=w321) -> ()  [unwired: 2 in, 2 out]
            n185 = property on="Rev/Fwd" class="Clust (strict)"("Visible"=w321) -> ()  [unwired: 2 in, 2 out]
            n186 = property on="Test Ring" class="Ring (strict)"("Visible"=w320) -> ()  [unwired: 2 in, 2 out]
            n187 = property on="Motor" class="Clust (strict)"("Visible"=w320) -> ()  [unwired: 2 in, 2 out]
          }
          frame "Analog Out", "Motor", "PWM" {
            w327 = FALSE ("Visible")
            n188 = case shown="\"Analog Out\"" w326 {
              tunnel: [1.0 ("Value") -1.0 ("Value") 0.0 ("Value")] -> w325
              tunnel: [255.0 ("Value") 1.0 ("Value") 5.0 ("Value")] -> w324
              tunnel: [128.0 ("Value") 0.0 ("Value") 0.0 ("Value")] -> w323
              tunnel: [64.0 ("Value") 0.5 ("Value") 1.0 ("Value")] -> w322
              frame "PWM" {
              }
              frame "Motor", Default {
              }
              frame "Analog Out" {
              }
            }
            n189 = property on="Test Slider" class="Slide (strict)"("Visible"=w327) -> ()  [unwired: 2 in, 2 out]
            n190 = property on="Test Ring" class="Ring (strict)"("Visible"=w327) -> ()  [unwired: 2 in, 2 out]
            n191 = property on="On/Off" class="Bool (strict)"("Visible"=w327) -> ()  [unwired: 2 in, 2 out]
            n192 = property on="Rev/Fwd" class="Clust (strict)"("Visible"=w327) -> ()  [unwired: 2 in, 2 out]
            n193 = property on="Motor" class="Clust (strict)"("Visible"=TRUE) -> ()  [unwired: 2 in, 2 out]
            n194 = property on="Value" class="Slide (strict)"("Value"=w323, "Scale.Minimum"=w325, "Scale.Maximum"=w324, "Scale.Increment"=w322) -> ()  [unwired: 2 in, 2 out]
          }
          frame "Servo" {
            w343 = FALSE ("Visible")
            n195 = call <vilib>:"NT Read Number.vi"("Name"=w345) -> ("Numeric"=w344:dbl)  [unwired: 9 in, 1 out]
            n196 = property on="Motor" class="Clust (strict)"("Visible"=w343) -> ()  [unwired: 2 in, 2 out]
            n197 = property on="Test Ring" class="Ring (strict)"("Visible"=w343) -> ()  [unwired: 2 in, 2 out]
            n198 = property on="On/Off" class="Bool (strict)"("Visible"=w343) -> ()  [unwired: 2 in, 2 out]
            n199 = property on="Rev/Fwd" class="Clust (strict)"("Visible"=w343) -> ()  [unwired: 2 in, 2 out]
            n200 = property on="Test Slider" class="Slide (strict)"("Visible"=TRUE, "Scale.Maximum"=170.0 ("Scale.Range:Maximum")) -> ()  [unwired: 2 in, 2 out]
            n201 = local write "Test Slider"(w344) -> ()
          }
          frame "Relay", "Solenoid" {
            w346 = FALSE ("Visible")
            n202 = property on="Motor" class="Clust (strict)"("Visible"=w346) -> ()  [unwired: 2 in, 2 out]
            n203 = property on="Test Slider" class="Slide (strict)"("Visible"=w346) -> ()  [unwired: 2 in, 2 out]
            n204 = property on="Test Ring" class="Ring (strict)"("Visible"=w346) -> ()  [unwired: 2 in, 2 out]
            n205 = Search and Replace String(input string=w347, search string="/Value  **", replace string="/Direction") -> (result string=w353:string)  [unwired: 5 in, 3 out]
            n206 = call <vilib>:"NT Read String.vi"("Name"=w353) -> ("String"=w351:string)  [unwired: 9 in, 1 out]
            n207 = Equal?(x="Both directions", y=w351) -> (x = y?=w349:bool)
            n208 = property on="Rev/Fwd" class="Clust (strict)"("Visible"=w349) -> ()  [unwired: 2 in, 2 out]
            n209 = Not(x=w349) -> (.not. x?=w350:bool)
            n210 = property on="On/Off" class="Bool (strict)"("Visible"=w350, "Caption.Text"=w348) -> ()  [unwired: 2 in, 2 out]
          }
          frame "Compressor", "Digital Out" {
            w356 = FALSE ("Visible")
            # "Get direction and finish"
            n211 = property on="Test Ring" class="Ring (strict)"("Visible"=w356) -> ()  [unwired: 2 in, 2 out]
            n212 = property on="Motor" class="Clust (strict)"("Visible"=w356) -> ()  [unwired: 2 in, 2 out]
            n213 = property on="Test Slider" class="Slide (strict)"("Visible"=w356) -> ()  [unwired: 2 in, 2 out]
            n214 = property on="Rev/Fwd" class="Clust (strict)"("Visible"=FALSE) -> ()  [unwired: 2 in, 2 out]
            n215 = property on="On/Off" class="Bool (strict)"("Visible"=TRUE, "Caption.Text"=w357) -> ()  [unwired: 2 in, 2 out]
          }
          frame "Camera" {
            n216 = call <vilib>:"Get Last Path Segment.vi"("String in"=w364) -> ("String out"=w365:string)  [unwired: 10 in]
            n217 = property on="Rev/Fwd" class="Clust (strict)"("Visible"=FALSE) -> ()  [unwired: 2 in, 2 out]
            n218 = case shown="\"White Balance  **\"" w365 {
              tunnel: w364 -> [w371 w380 w389 w398 w407 _ w413]
              tunnel: w363 -> [w369 w377 w386 w395 w404 _ _]
              frame "Size  **" {
                n219 = Index Array(array=w369) -> (element=w368:cluster{string[]})  [unwired: 1 in]
                n220 = call <vilib>:"NT Read String.vi"("Name"=w371) -> ("String"=w370:string)  [unwired: 9 in, 1 out]
                n221 = property on="Test Slider" class="Slide (strict)"("Visible"=FALSE) -> ()  [unwired: 2 in, 2 out]
                n222 = property on="Test Ring" class="Ring (strict)"("Visible"=TRUE) -> ()  [unwired: 2 in, 2 out]
                n223 = Unbundle(w368) -> (w366:string[])
                n224 = Match First String(2:w366, 3:w370) -> (0:w367:i32)  [unwired: 1 out]
                n225 = property on="Test Ring" class="Ring (strict)"("Value"=w367, "Strings []"=w366) -> ()  [unwired: 2 in, 2 out]
              }
              frame "White Balance  **" {
                n226 = call <vilib>:"NT Read String.vi"("Name"=w380) -> ("String"=w379:string)  [unwired: 9 in, 1 out]
                n227 = Index Array(array=w377, index=1) -> (element=w378:cluster{string[]})
                n228 = property on="Test Slider" class="Slide (strict)"("Visible"=FALSE) -> ()  [unwired: 2 in, 2 out]
                n229 = property on="Test Ring" class="Ring (strict)"("Visible"=TRUE) -> ()  [unwired: 2 in, 2 out]
                n230 = Unbundle(w378) -> (w375:string[])
                n231 = Match First String(2:w375, 3:w379) -> (0:w374:i32)  [unwired: 1 out]
                n232 = property on="Test Ring" class="Ring (strict)"("Value"=w374, "Strings []"=w375) -> ()  [unwired: 2 in, 2 out]
              }
              frame "Exposure  **" {
                n233 = call <vilib>:"NT Read String.vi"("Name"=w389) -> ("String"=w388:string)  [unwired: 9 in, 1 out]
                n234 = Index Array(array=w386, index=2) -> (element=w387:cluster{string[]})
                n235 = property on="Test Slider" class="Slide (strict)"("Visible"=FALSE) -> ()  [unwired: 2 in, 2 out]
                n236 = property on="Test Ring" class="Ring (strict)"("Visible"=TRUE) -> ()  [unwired: 2 in, 2 out]
                n237 = Unbundle(w387) -> (w383:string[])
                n238 = Match First String(2:w383, 3:w388) -> (0:w384:i32)  [unwired: 1 out]
                n239 = property on="Test Ring" class="Ring (strict)"("Value"=w384, "Strings []"=w383) -> ()  [unwired: 2 in, 2 out]
              }
              frame "Exposure Priority  **" {
                n240 = call <vilib>:"NT Read String.vi"("Name"=w398) -> ("String"=w397:string)  [unwired: 9 in, 1 out]
                n241 = Index Array(array=w395, index=3) -> (element=w396:cluster{string[]})
                n242 = property on="Test Slider" class="Slide (strict)"("Visible"=FALSE) -> ()  [unwired: 2 in, 2 out]
                n243 = property on="Test Ring" class="Ring (strict)"("Visible"=TRUE) -> ()  [unwired: 2 in, 2 out]
                n244 = Unbundle(w396) -> (w392:string[])
                n245 = Match First String(2:w392, 3:w397) -> (0:w393:i32)  [unwired: 1 out]
                n246 = property on="Test Ring" class="Ring (strict)"("Value"=w393, "Strings []"=w392) -> ()  [unwired: 2 in, 2 out]
              }
              frame "Color Enable  **" {
                n247 = call <vilib>:"NT Read String.vi"("Name"=w407) -> ("String"=w406:string)  [unwired: 9 in, 1 out]
                n248 = Index Array(array=w404, index=4) -> (element=w405:cluster{string[]})
                n249 = property on="Test Slider" class="Slide (strict)"("Visible"=FALSE) -> ()  [unwired: 2 in, 2 out]
                n250 = property on="Test Ring" class="Ring (strict)"("Visible"=TRUE) -> ()  [unwired: 2 in, 2 out]
                n251 = Unbundle(w405) -> (w401:string[])
                n252 = Match First String(2:w401, 3:w406) -> (0:w402:i32)  [unwired: 1 out]
                n253 = property on="Test Ring" class="Ring (strict)"("Value"=w402, "Strings []"=w401) -> ()  [unwired: 2 in, 2 out]
              }
              frame Default {
                n254 = property on="Test Slider" class="Slide (strict)"("Visible"=FALSE) -> ()  [unwired: 2 in, 2 out]
                n255 = property on="Test Ring" class="Ring (strict)"("Visible"=FALSE) -> ()  [unwired: 2 in, 2 out]
              }
              frame "Brightness  **", "Color Level  **", "Compression  **", "FPS  **", "Sharpness  **" {
                n256 = call <vilib>:"NT Read Number.vi"("Name"=w413) -> ("Numeric"=w412:dbl)  [unwired: 9 in, 1 out]
                n257 = property on="Test Ring" class="Ring (strict)"("Visible"=FALSE) -> ()  [unwired: 2 in, 2 out]
                n258 = property on="Test Slider" class="Slide (strict)"("Visible"=TRUE, "Scale.Maximum"=100.0 ("Scale.Range:Maximum")) -> ()  [unwired: 2 in, 2 out]
                n259 = local write "Test Slider"(w412) -> ()
              }
            }
            n260 = property on="Motor" class="Clust (strict)"("Visible"=FALSE) -> ()  [unwired: 2 in, 2 out]
            n261 = property on="On/Off" class="Bool (strict)"("Visible"=FALSE) -> ()  [unwired: 2 in, 2 out]
          }
        }
      }
      event "Test Name": Mouse Enter {
        # "Populate the ring with the list of tests"
        n262 = event-data() -> ()  [unwired: 1 in, 1 out]
        n263 = call <vilib>:"NT Read String Array.vi"("Name"="/TestMode/TestList") -> ("String Array"=w421:string[])  [unwired: 9 in, 1 out]
        n264 = Build Array (concatenate)("Select the test to run...", w421) -> (w420:string[])
        n265 = property on="Test Name" class="Ring (strict)"("Strings []"=w420) -> ()  [unwired: 2 in, 2 out]
      }
      event "Test Name": Value Change {
        w423 = FALSE ("Visible")
        # "Tell the robot the test name to run"
        n266 = event-data() -> ("NewVal"=w427:u16)  [unwired: 1 in]
        n267 = property on="Test Name" class="Ring (strict)"() -> ("Strings []"=w428:string[])  [unwired: 2 in, 2 out]
        n268 = property on="Progress" class="Clust (strict)"("Visible"=TRUE) -> ()  [unwired: 2 in, 2 out]
        n269 = local write "Progress"(T10 {"Test Progress"=0, "Test Progress Text"=""} ("Progress")) -> ()
        n270 = property on="Test Ring" class="Ring (strict)"("Visible"=w423) -> ()  [unwired: 2 in, 2 out]
        n271 = property on="Motor" class="Clust (strict)"("Visible"=w423) -> ()  [unwired: 2 in, 2 out]
        n272 = property on="Test Slider" class="Slide (strict)"("Visible"=w423) -> ()  [unwired: 2 in, 2 out]
        n273 = property on="On/Off" class="Bool (strict)"("Visible"=w423) -> ()  [unwired: 2 in, 2 out]
        n274 = property on="Rev/Fwd" class="Clust (strict)"("Visible"=w423) -> ()  [unwired: 2 in, 2 out]
        n275 = Index Array(array=w428, index=w427) -> (element=w426:string)
        n276 = call <vilib>:"NT Write String.vi"("String"=w426, "Name"="/TestMode/TestName") -> ()  [unwired: 9 in, 1 out]
      }
      event "Select Auto": Mouse Enter {
        # "Populate the combo box with the list of autonomous options"
        n277 = event-data() -> ()  [unwired: 1 in, 1 out]
        n278 = call <vilib>:"NT Read String Array.vi"("Name"="Auto List") -> ("String Array"=w430:string[])  [unwired: 9 in, 1 out]
        n279 = property on="Select Auto" class="CmbBox"("Strings[]"=w430) -> ()  [unwired: 2 in, 2 out]
      }
      event "Select Auto": Value Change {
        # "User modified the Auto Selection. Write to NT variable so robot knows."
        n280 = event-data() -> ("NewVal"=w433:string)  [unwired: 1 in]
        n281 = call <vilib>:"NT Write String.vi"("String"=w433, "Name"="Auto Selector") -> ()  [unwired: 9 in, 1 out]
      }
      event "Command Selection": Value Change {
        # "Get the params and show in table"
        n282 = event-data() -> ("NewVal"=w439:i32)  [unwired: 1 in]
        n283 = property on="Command Selection" class="MCListbox (strict)"() -> ("ItemNames"=w437:string[][])  [unwired: 2 in, 2 out]
        n284 = call <vilib>:"WPI_DashboardUpdate Command Params.vi"("NewVal"=w439, "Commands"=w437, "Param Tbl"=w438) -> ()  [unwired: 8 in, 1 out]
      }
      event "Execute Command": Value Change {
        # "Started one, Unique ID holds\nresponse"
        n285 = event-data() -> ()  [unwired: 1 in, 1 out]
        n286 = property on="Command Selection" class="MCListbox (strict)"() -> ("ItemNames"=w450:string[][])  [unwired: 2 in, 2 out]
        n287 = Index Array(array=w450, index (row)="Command Selection", index (col)=0) -> (element=w448:string)
        n288 = call <vilib>:"Invoke Commands.vi"("Command Params"="Command Params", "Function Name"=w448) -> ("Params"=w444:u8, "Started"=w443:bool)  [unwired: 7 in, 1 out]
        n289 = Array Subset(array="Command Params", length (row)=w444) -> (w445:string[][])  [unwired: 3 in]
        n290 = Select(t="Executing" ("Cmd Status"), s=w443, f="" ("Cmd Status")) -> (s? t:f=→"Cmd Status":string)
      }
      event "Command Selection": Double Click {
        n291 = event-data() -> ("Row"=w458:i32)  [unwired: 1 in]
        n292 = property on="Command Selection" class="MCListbox (strict)"() -> ("ItemNames"=w461:string[][])  [unwired: 2 in, 2 out]
        n293 = local read "Command Params"() -> (w457:string[][])
        n294 = Index Array(array=w461, index (row)=w458, index (col)=0) -> (element=w459:string)
        n295 = call <vilib>:"Invoke Commands.vi"("Command Params"=w457, "Function Name"=w459) -> ("Params"=w456:u8, "Started"=w451:bool)  [unwired: 7 in, 1 out]
        n296 = Array Subset(array=w457, length (row)=w456) -> (w455:string[][])  [unwired: 3 in]
        n297 = Select(t="Executing" ("Cmd Status"), s=w451, f="" ("Cmd Status")) -> (s? t:f=w452:string)
        n298 = local write "Cmd Status"(w452) -> ()
      }
      event "CheckList": Double Click {
        # "Shift clears all"
        # "Update symbols on the listbox"
        n299 = event-data() -> ("PlatMods.Shift"=w463:bool, "Row"=w465:i32)  [unwired: 1 in]
        n300 = case shown="True" w463 {
          tunnel: w465 -> [w469 _]
          tunnel: 1 -> [w468 _]
          frame False {
            n301 = property on="CheckList" class="LstBox (strict)"() -> ("Item Symbols"=w467:i32[])  [unwired: 2 in, 2 out]
            n302 = Replace Array Subset(array=w467, new element=w468, index=w469) -> (w466:i32[])
            n303 = property on="CheckList" class="LstBox (strict)"("Item Symbols"=w466) -> ()  [unwired: 2 in, 2 out]
          }
          frame True {
            w470 = 0 ("Top Row")
            n304 = property on="CheckList" class="LstBox (strict)"() -> ("Number of Rows"=w472:u32)  [unwired: 2 in, 2 out]
            n305 = Initialize Array(0, w472) -> (w471:i32[])
            n306 = property on="CheckList" class="LstBox (strict)"("Top Row"=w470, "Value"=w470, "Item Symbols"=w471) -> ()  [unwired: 2 in, 2 out]
          }
        }
      }
      event "CheckList": Key Down {
        # "Update symbols on the listbox\nLeft and right keys check and uncheck"
        n307 = event-data() -> ("VKey"=w476:T23)  [unwired: 1 in]
        n308 = case shown="\"Left\", \"Right\"" w476 {
          selector: w476 -> [w481 _]
          tunnel: eventvkey."Left" ("VKey") -> [w479 _]
          frame "Left", "Right" {
            n309 = Equal?(x=w479, y=w481) -> (x = y?=w480:bool)
            n310 = Select(t=0, s=w480, f=1) -> (s? t:f=w482:i32)
            n311 = property on="CheckList" class="LstBox (strict)"() -> ("Item Symbols"=w485:i32[])  [unwired: 2 in, 2 out]
            n312 = Replace Array Subset(array=w485, new element=w482, index="CheckList") -> (w484:i32[])
            n313 = property on="CheckList" class="LstBox (strict)"("Item Symbols"=w484) -> ()  [unwired: 2 in, 2 out]
          }
          frame Default {
          }
        }
      }
      event "Motor.Enable": Value Change {
        # "When the test mode otor enable helper is set, update that\ntree row item's value"
        n314 = event-data() -> ("NewVal"=w491:bool)  [unwired: 1 in]
        n315 = Unbundle("Motor") -> ("Value"=w490:dbl)  [unwired: 1 out]
        n316 = Select(t=w490, s=w491, f=0.0) -> (s? t:f=w488:dbl)
        n317 = call <vilib>:"NT Write Number.vi"("Numeric"=w488, "Name"=w487) -> ()  [unwired: 9 in, 1 out]
      }
      event "Test Slider": Value Change {
        # "When the test mode slider helper is set, update that\ntree row item's value"
        n318 = event-data() -> ("NewVal"=w494:dbl)  [unwired: 1 in]
        n319 = call <vilib>:"NT Write Number.vi"("Numeric"=w494, "Name"=w495) -> ()  [unwired: 9 in, 1 out]
      }
      event "On/Off": Value Change {
        # "When the test mode on/off helper value is set, update that\ntree row item's value"
        n320 = event-data() -> ("NewVal"=w499:bool)  [unwired: 1 in]
        n321 = Boolean To (0,1)(Boolean=w499) -> (0, 1=w498:i16)
        n322 = call <vilib>:"NT Write Number.vi"("Numeric"=w498, "Name"=w497) -> ()  [unwired: 9 in, 1 out]
      }
      event "Rev/Fwd": Value Change {
        # "When the test mode helper value for relays is set, update that\ntree row item's value"
        n323 = event-data() -> ("NewVal.Forward"=w507:bool, "NewVal.Reverse"=w506:bool)  [unwired: 1 in]
        n324 = Boolean To (0,1)(Boolean=w507) -> (0, 1=w503:i16)
        n325 = Boolean To (0,1)(Boolean=w506) -> (0, 1=w505:i16)
        n326 = Negate(x=w505) -> (-x=w504:i16)
        n327 = Add(x=w503, y=w504) -> (x+y=w502:i16)
        n328 = call <vilib>:"NT Write Number.vi"("Numeric"=w502, "Name"=w501) -> ()  [unwired: 9 in, 1 out]
      }
      event "Test Ring": Value Change {
        # "When a test mode helper value is selected from the ring,\nset the tree item's variable to the string value"
        n329 = event-data() -> ("NewVal"=w511:u16)  [unwired: 1 in]
        n330 = property on="Test Ring" class="Ring (strict)"() -> ("Strings []"=w512:string[])  [unwired: 2 in, 2 out]
        n331 = Index Array(array=w512, index=w511) -> (element=w510:string)
        n332 = call <vilib>:"NT Write String.vi"("String"=w510, "Name"=w509) -> ()  [unwired: 9 in, 1 out]
      }
      event "Rec Mode": Value Change {
        # "Update globals for recording mode and path to read log from.\nClear when logging and let NetworkTables set path for vision to\nuse."
        n333 = event-data() -> ("NewVal"=w523:enum32{"Stop", "Record", "Playback"})  [unwired: 1 in]
        n334 = global write "WPI_DashboardLogging Global.vi" "Logging Filename"(path "") -> ()
        n335 = global write "WPI_DashboardLogging Global.vi" "Recording"(w523) -> ()
        n336 = call <vilib>:"WPI_DashboardNT Log FieldName Cache.vi"("Operation"=enum16{"Lookup/Add", "Index", "Clear"}."Clear") -> ()  [unwired: 8 in, 3 out]
        n337 = case shown="\"Playback\"" w523 {
          tunnel: w522 -> [_ w525 w534]
          tunnel: [_ _ w533] -> w520
          tunnel: [_ _ w532] -> _
          tunnel: w518 -> [_ _ w530]
          tunnel: cluster{i32, i32} {-250, 170} -> [_ _ w529]
          tunnel: [_ _ T24 {"Image Size"=TRUE, "Image Type"=TRUE, "Pixel Value"=TRUE, "ROI Information"=TRUE, "Zoom Factor"=FALSE} ("Image Information Shown:All Elements")] -> w516
          tunnel: [_ _ TRUE ("Zoom Factor")] -> w515
          tunnel: w514 -> [_ _ w526]
          frame Default {
          }
          frame "Stop", "Record" {
            # "Place Window too"
            n338 = invoke class="VI" method="FP.Close"(reference=w525) -> (reference out=w524:refnum<vi>)  [unwired: 2 in, 2 out]
            n339 = invoke class="VI" method="Abort VI"(reference=w524) -> ()  [unwired: 2 in, 3 out]
          }
          frame "Playback" {
            n340 = call "Open Playback Panel.vi"("Offset"=w529, "DB VI Ref"=w530, "Playback in"=w534) -> ("Playback out"=w531:refnum<vi>)  [unwired: 8 in]
            n341 = register-events(w531, w526) -> (reference out=w533:refnum<event-registration>, error out=w532:errorcluster)  [unwired: 2 in]
          }
        }
        n342 = property on="Camera Image" class="ImageControl"("Image Information Shown"=w516, "Image Information Visible"=w515) -> ()  [unwired: 2 in, 2 out]
      }
      event Panel Close {
        w536 = enum32{"Stop", "Record", "Playback"}."Stop" ("Rec Mode")
        # "Playback window has been closed, abort"
        n343 = event-data() -> ()  [unwired: 1 in, 4 out]
        n344 = local write "Rec Mode"(w536) -> ()
        n345 = global write "WPI_DashboardLogging Global.vi" "Recording"(w536) -> ()
      }
      event Panel Close {
        # "Abort playback window and ourself"
        n346 = event-data() -> ()  [unwired: 1 in, 4 out]
        n347 = invoke class="VI" method="FP.Close"(reference=w540) -> (reference out=w539:refnum<vi>)  [unwired: 2 in, 2 out]
        n348 = invoke class="VI" method="Abort VI"(reference=w539) -> (error out=w538:errorcluster)  [unwired: 2 in, 2 out]
        n349 = invoke class="VI" method="Abort VI"(error in=w538) -> ()  [unwired: 2 in, 3 out]
      }
      event User Event {
        n350 = event-data() -> ("IDs"=w547:cluster{"RPC field ID":u16, "Unique ID":u16}, "String"=w546:string)  [unwired: 1 in]
        n351 = local write "Cmd Status"("" ("Cmd Status")) -> ()
        n352 = Bundle("IDs"=w547, "String"=w546) -> (w545:T12)  [unwired: 1 in]
        n353 = call <vilib>:"Retrieve RPC Response.vi"("RPC Response"=w545) -> ("Output"=w543:string[][])  [unwired: 10 in]
        n354 = Build Array (concatenate)(w541, w543) -> (w542:string[][])
        n355 = local write "Command Params"(w542) -> ()
      }
      event "Tree": Double Click {
        n356 = event-data() -> ("PlatMods"=w551:T27, "Tag"=w550:string)  [unwired: 1 in]
        n357 = Unbundle(w551) -> ("Shift"=w549:bool)  [unwired: 4 out]
        n358 = Not(x=w549) -> (.not. x?=w548:bool)
        n359 = call <vilib>:"NT Update Persistence.vi"("Persistence"=w548, "Name"=w550) -> ()  [unwired: 9 in, 1 out]
      }
    }
  }
